vi "Cell Enable.vi"(7 "Box ID":u8=1, 8 "error in (no error)":errorcluster, 9 "Enable":bool, 10 "Channel":u16=1 min=1 max=12 step=1, 11 "CAN in":refnum<class "XNET_BS120x.lvclass">) -> (0 "error out":errorcluster, 3 "CAN out":refnum<class "XNET_BS120x.lvclass">)   [LabVIEW 2021, in "BS120x Driver.lvlib" / "XNET_BS120x.lvclass"]
uses:
  XNET_BS120x.lvclass
  BS120x.lvclass
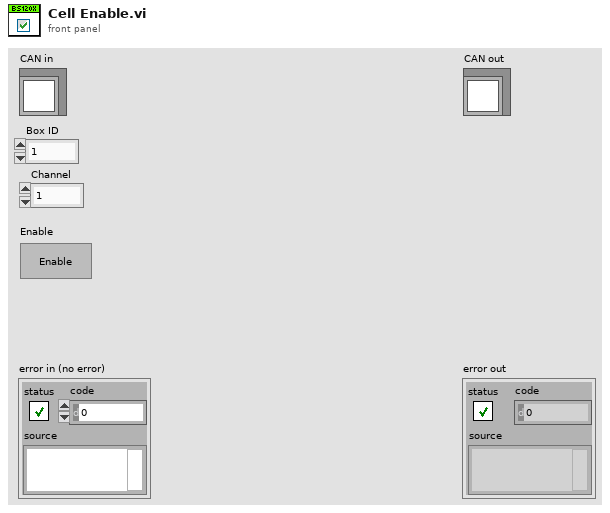
[diagram p1: front panel]
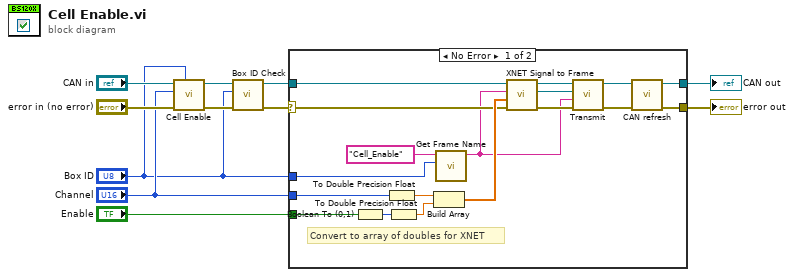
[diagram p0: block diagram]
diagram:
  n1 = call-parent "Cell Enable.vi"("Box ID"="Box ID", "error in (no error)"="error in (no error)", "Channel"="Channel", "BS120x in"="CAN in") -> ("error out"=w4:errorcluster, "BS120x out"=w5:refnum<class "XNET_BS120x.lvclass">)  [unwired: 6 in]
  n2 = call "Box ID Check.vi"("error in (no error)"=w4, "Box ID"="Box ID", "CAN in"=w5) -> ("error out"=w6:errorcluster, "CAN out"=w7:refnum<class "XNET_BS120x.lvclass">)  [unwired: 7 in]
  n3 = case shown="No Error" w6 {
    selector: w6 -> [w13 w31]
    tunnel: "Channel" -> [w26 _]
    tunnel: "Enable" -> [w25 _]
    tunnel: [w19 w31] -> w10
    tunnel: [w17 w30] -> w9
    tunnel: w7 -> [w15 w30]
    tunnel: "Box ID" -> [w14 _]
    frame No Error {
      # "Convert to array of doubles for XNET"
      n4 = Boolean To (0,1)(Boolean=w25) -> (0, 1=w29:i16)
      n5 = To Double Precision Float(number=w26) -> (double precision float=w27:dbl)
      n6 = To Double Precision Float(number=w29) -> (double precision float=w28:dbl)
      n7 = Build Array(w27, w28) -> (w24:dbl[])
      n8 = call "Get Frame Name.vi"("Box ID"=w14, "Frame Name"="Cell_Enable" ("Frame")) -> ("Frame Name out"=w12:string)  [unwired: 9 in]
      n9 = call "XNET Signal to Frame.vi"("error in (no error)"=w13, "Data Array"=w24, "Frame"=w12, "CAN in"=w15) -> ("error out"=w21:errorcluster, "Data"=w22:refnum<class "XNET Data.lvclass">, "CAN out"=w23:refnum<class "XNET_BS120x.lvclass">)  [unwired: 5 in]
      n10 = call "Transmit.vi"("error in (no error)"=w21, "Frame"=w12, "Data in"=w22, "CAN in"=w23) -> ("error out"=w20:errorcluster, "CAN out"=w18:refnum<class "XNET_BS120x.lvclass">)  [unwired: 6 in]
      n11 = call "CAN refresh.vi"("error in (no error)"=w20, "CAN in"=w18) -> ("error out"=w19:errorcluster, "CAN out"=w17:refnum<class "XNET_BS120x.lvclass">)  [unwired: 8 in]
    }
    frame Error {
    }
  }
  "error out" <- w10
  "CAN out" <- w9
